vi "Initialize Channel Group Channels.vi"(8 "error in":errorcluster, 9 "default decimation value":i32, 11 "channel group reference in":T1 format="%.0x") -> (0 "error out":errorcluster, 3 "channel group reference out":T1 format="%.0x")   [LabVIEW 2027, in "Embedded Data Logger Scripting.lvlib"]
uses:
  Embedded Data Logger Scripting.lvlib
  <vilib>/NI VeriStand/Custom Device API/Custom Device Item Ref.ctl
  <vilib>/NI VeriStand/Custom Device API/Custom Device Channel.ctl
  <vilib>/NI VeriStand/Custom Device API/Custom Device Channel Type.ctl
  Shared/Constants.vi
  <vilib>/NI VeriStand/Custom Device API/Custom Device API.lvlib
  Shared/Embedded Data Logger Shared.lvlib
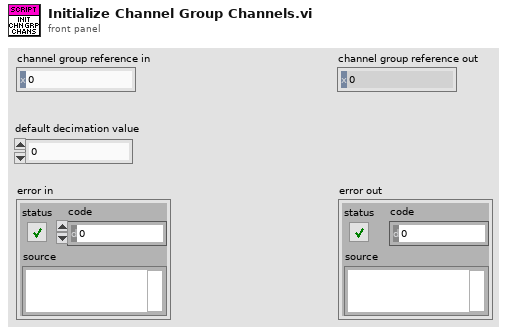
[diagram p1: front panel]
types:
  T1 = typedef "Custom Device API.lvlib/Custom Device Item Ref.ctl" = u64
  T2 = typedef "Custom Device API.lvlib/Custom Device Channel.ctl" = cluster{"Type":T3, "Units":string, "Default Value":dbl, "Faultable":bool, "Scalable":bool}
  T3 = typedef "Custom Device API.lvlib/Custom Device Channel Type.ctl" = enum16{"Input", "Output"}
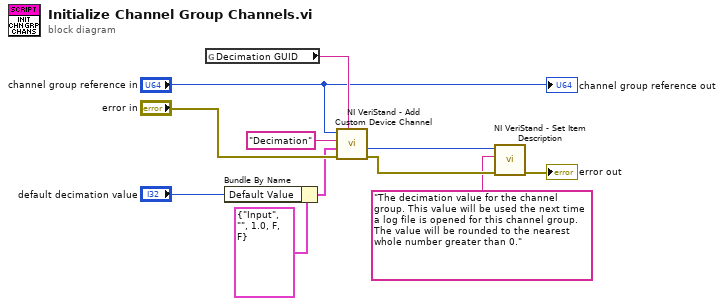
[diagram p0: block diagram]
diagram:
  n1 = global read "Constants.vi" "Decimation GUID"() -> (w8:string)
  n2 = Bundle By Name(cluster=T2 {"Type"=enum."Input", "Units"="", "Default Value"=1.0, "Faultable"=FALSE, "Scalable"=FALSE} ("Channel"), "Default Value"="default decimation value") -> (w2:T2)
  n3 = call <vilib>:"NI VeriStand - Add Custom Device Channel.vi"("GUID (Default Channel)"=w8, "error in (no error)"="error in", "Channel"=w2, "Channel Name"="Decimation", "Parent Ref in"="channel group reference in") -> ("error out"=w10:errorcluster, "Channel Ref"=w9:T1)  [unwired: 3 in, 2 out]
  n4 = call <vilib>:"NI VeriStand - Set Item Description.vi"("error in (no error)"=w10, "Description"="The decimation value for the channel group. This value will be used the next time a log file is opened for this channel group. The value will be rounded to the nearest whole number greater than 0." ("String"), "Item Ref in"=w9) -> ("error out"=→"error out":errorcluster)  [unwired: 6 in, 2 out]
  "channel group reference out" <- "channel group reference in"
